vi "Pre Launch Init.vi"(11 "NI in":refnum<class "NI.lvclass">) -> (0 "error out":errorcluster, 3 "NI out":refnum<class "NI.lvclass">)   [LabVIEW 2021, in "NI.lvlib" / "NI.lvclass"]
doc: "(<B>Filename</B>: Actor Framework.lvlib:Actor.lvclass:Pre Launch Init.vi)\n\nDefines behavior that occurs after the Launch Nested Actor method is invoked but before the actor's Actor Core method begins running.\n\nBy default, this method does nothing. A descendant class may override it to define behavior."
uses:
  NI.lvclass
  Channel Connection.ctl
  Utilities/RWC_Actions.ctl
  NI.lvclass/NI.ctl
  <vilib>/ActorFramework/Actor/Actor.lvclass
panel:
  in  "Inner parameters":T2
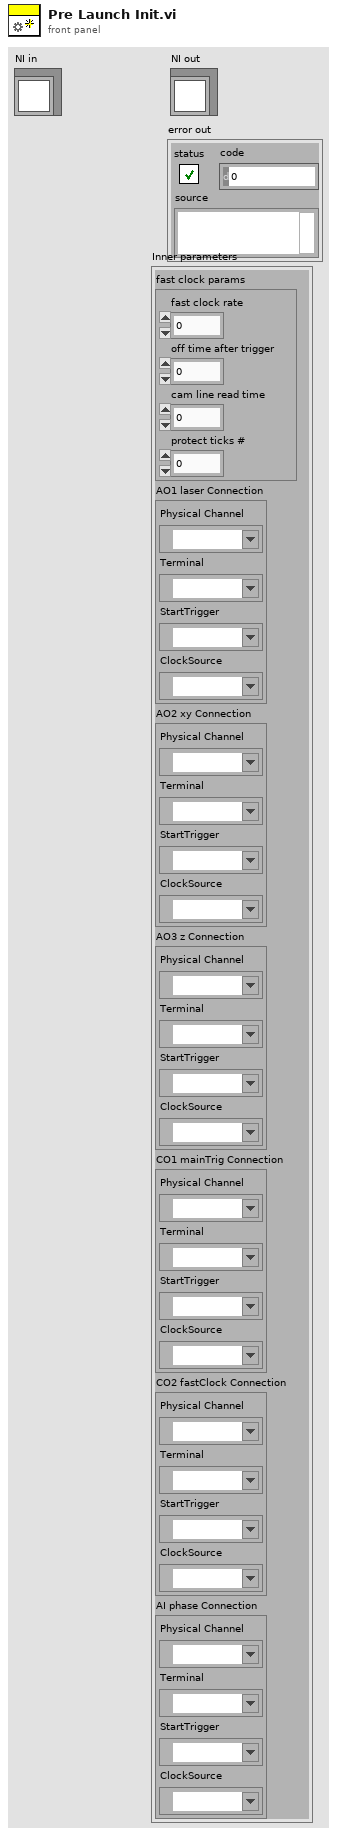
[diagram p1: front panel]
types:
  T1 = typedef "NI.lvlib/NI.lvclass/Channel Connection.ctl" = cluster{"Physical Channel":tag, "Terminal":tag, "StartTrigger":tag, "ClockSource":tag}
  T2 = cluster{"fast clock params":cluster{"fast clock rate":dbl, "off time after trigger":dbl, "cam line read time":dbl, "protect ticks #":dbl}, "AO1 laser Connection":T1, "AO2 xy Connection":T1, "AO3 z Connection":T1, "CO1 mainTrig Connection":T1, "CO2 fastClock Connection":T1, "AI phase Connection":T1}
  T3 = typedef "RWC_Actions.ctl" = enum16{"Read", "Write", "Read and Create"}
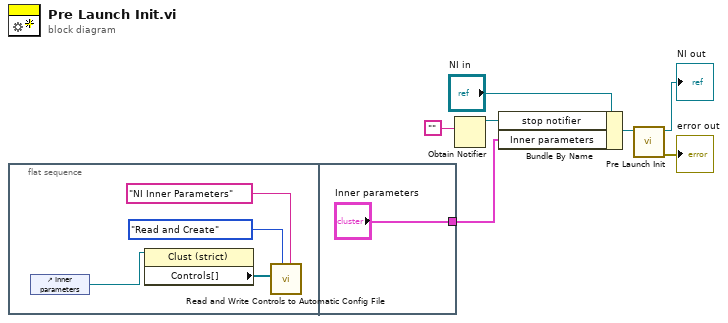
[diagram p0: block diagram]
diagram:
  n1 = flat-sequence {
    tunnel: ["Inner parameters"] -> w1
    frame #0 {
      n2 = control-ref of="Inner parameters"() -> (w8:refnum<vi>)
      n3 = property class="Clust (strict)"(reference=w8) -> ("Controls[]"=w9:refnum<vi>[])  [unwired: 1 in, 2 out]
      n4 = call "Read and Write Controls to Automatic Config File.vi"("file name"="NI Inner Parameters" ("section (optional)"), "Action"=RWC_Actions."Read and Create", "Control References"=w9) -> ()  [unwired: 8 in, 1 out]
    }
    frame #1 {
    }
  }
  n5 = Obtain Notifier(notification data type="") -> (notifier out=w5:refnum<notifier>)  [unwired: 3 in, 2 out]
  n6 = Bundle By Name(cluster="NI in", "stop notifier"=w5, "Inner parameters"=w1) -> (w3:refnum<class "NI.lvclass">)
  n7 = call-parent "Pre Launch Init.vi"("Actor in"=w3) -> ("error out"=→"error out":errorcluster, "Actor out"=→"NI out":refnum<class "NI.lvclass">)  [unwired: 9 in]
